vi "Common Function.vi"(6 "exit sig":refnum<k4>, 11 "gController in":refnum<class "gController.lvclass">) -> ()   [LabVIEW 2017, in "Controller.lvlib" / "gController.lvclass"]
uses:
  gController.lvclass
  C:/Program Files (x86)/National Instruments/LabVIEW 2017/vi.lib/MSR Consulting, LLC/General Reuse/SuperActor/SuperActor.lvclass
  C:/Program Files (x86)/National Instruments/LabVIEW 2017/vi.lib/ActorFramework/Actor/Actor.lvclass
  <vilib>/Platform/TimedLoop/XDataNode/timing_clust.ctl
  <vilib>/Platform/TimedLoop/XDataNode/nitl_modes.ctl
  <vilib>/Platform/TimedLoop/XDataNode/wakeup.ctl
  gController.lvclass/gController.ctl
  <vilib>/MSR Consulting, LLC/General Reuse/SuperActor/SuperActor.lvclass/SuperActor.ctl
  <vilib>/ActorFramework/Actor/Actor.lvclass/Actor.ctl
  <vilib>/ActorFramework/Message Enqueuer/Message Enqueuer.lvclass/Message Enqueuer.ctl
  <vilib>/MSR Consulting, LLC/General Reuse/Data/Data.lvclass/Data.ctl
  Messages/Update Controller Data MSG/Update gController Data MSG.lvclass
  C:/Program Files (x86)/National Instruments/LabVIEW 2017/vi.lib/MSR Consulting, LLC/General Reuse/Generic Update Data MSG/Generic Update Data MSG.lvclass
  C:/Program Files (x86)/National Instruments/LabVIEW 2017/vi.lib/ActorFramework/Message/Message.lvclass
  Data/SOAP Data.lvclass/SOAP Data.ctl
  <vilib>/MSR Consulting, LLC/General Reuse/Generic Update Data MSG/Generic Update Data MSG.lvclass/Generic Update Data MSG.ctl
  Data/Write temperatures.vi
  Data/Write interlock.vi
  Data/Read message_data.vi
  <vilib>/MSR Consulting, LLC/General Reuse/Generic Update Data MSG/Write Data.vi
  <vilib>/MSR Consulting, LLC/General Reuse/Generic Update Data MSG/Write ID.vi
  Read FPGA Session.vi
  <vilib>/MSR Consulting, LLC/General Reuse/SuperActor/Read Log Session.vi
  <vilib>/MSR Consulting, LLC/General Reuse/SuperActor/Read CVT Session.vi
  <vilib>/MSR Consulting, LLC/General Reuse/Data/Write write time.vi
  <vilib>/ActorFramework/Message Enqueuer/Init from Existing Queue.vi
  Session/Raw FPGA/FPGA Session.lvclass
  C:/Program Files (x86)/National Instruments/LabVIEW 2017/vi.lib/MSR Consulting, LLC/General Reuse/Session APIs/_Session Fwk/Session - Root.lvclass
  Data/SOAP Data.lvclass
  C:/Program Files (x86)/National Instruments/LabVIEW 2017/vi.lib/MSR Consulting, LLC/General Reuse/Data/Data.lvclass
  Global DO.vi
  <vilib>/Utility/error.llb/Error Cluster From Error Code.vi
  <vilib>/rvi/errors/niLvFpgaAdjustHostInterfaceError.vi
  <vilib>/MSR Consulting, LLC/General Reuse/Data/Write measTime.vi
  <vilib>/ActorFramework/Message Priority Queue/Priority Enqueue.vi
  <vilib>/MSR Consulting, LLC/General Reuse/Session APIs/_Session Fwk/Session - Root.lvclass
  <vilib>/ActorFramework/Message Enqueuer/Message Enqueuer.lvclass
  <vilib>/Platform/TimedLoop/XDataNode/XDataNode.xnode
  Data/Heater Data/Heater Data.lvclass
  <vilib>/rvi/interface/nirviReadWriteControl/nirviReadWriteControl.xnode
  FPGA Ref.ctl
  FPGA Bitfiles/server.lvbitx
  <vilib>/MSR Consulting, LLC/General Reuse/SuperActor/SuperActor.lvclass
  <vilib>/Platform/TimedLoop/XDataNode/XDNodeRunTimeDep.lvlib
  <vilib>/MSR Consulting, LLC/General Reuse/Session APIs/Session Log/System Log.lvclass
  <vilib>/ActorFramework/Actor/Actor.lvclass
  NiFpgaLv.dll
  <vilib>/MSR Consulting, LLC/General Reuse/Session APIs/CVT/CVT.lvclass
panel:
  out "Iteration Duration":i64
  out "exceeds_dead_line":bool
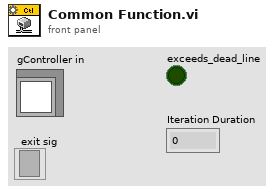
[diagram p1: front panel]
types:
  T1 = typedef "Session - Root.lvclass/Session Handle.ctl" = refnum<data-value>
  T2 = typedef "FPGA Ref.ctl" = refnum<k20>
  T3 = typedef "XDNodeRunTimeDep.lvlib/timing_clust.ctl" = cluster{"Expected End [f-1]":u64, "Actual End [f-1]":u64, "Finished Late? [f-1]":bool, "Expected End [i-1]":u64, "Actual End [i-1]":u64, "Finished Late? [i-1]":bool, "Expected Start [i]":u64, "Actual Start [i]":u64, "Expected Start [f]":u64, "Actual Start [f]":u64, "Source Name":string, "Structure Name":string, "Period":i64, "Deadline":i64, "Offset":i64, "Start":i64, "Priority":i32, "Timeout":i32, "Mode":T4, "Wakeup Reason":T5, "Error":errorcluster, "Source Type":string, "Secondary Source Type":string, "Global End Time":u64, "Global Start Time":u64, "Frame Duration":u64, "Iteration Duration":u64, "Assigned CPU":i32, "I/O Scan Engine Mode":u32}
  T4 = typedef "XDNodeRunTimeDep.lvlib/nitl_modes.ctl" = enum32{"No Change", "Process missed periods, maintain original phase", "Discard missed periods, maintain original phase", "Process missed periods, ignore original phase", "Discard missed periods, ignore original phase"}
  T5 = typedef "XDNodeRunTimeDep.lvlib/wakeup.ctl" = enum32{"Normal", "Aborted", "Asynchronous wakeup", "Timing source error", "Timed loop error", "Timeout"}
  T6 = cluster{"PAS Cell 1 Temperature":fxp<+/-,24,-2>, "PAS Cell 2 Temperature":fxp<+/-,24,-2>, "PAS Laser Head 1 Temperature":fxp<+/-,24,-2>, "PAS Laser Head 2 Temperature":fxp<+/-,24,-2>, "CRD Laser Head Temperature":fxp<+/-,24,-2>, "Box In Temperature":fxp<+/-,24,-2>, "Box Exit Temperature":fxp<+/-,24,-2>, "CRD Heater Temperature":fxp<+/-,24,-2>, "CJC":fxp<+/-,24,-2>, "Autozero":fxp<+/-,24,-2>}
  T7 = cluster{"PAS Cell 1 Temperature":dbl, "PAS Cell 2 Temperature":dbl, "PAS Laser Head 1 Temperature":dbl, "PAS Laser Head 2 Temperature":dbl, "CRD Laser Head Temperature":dbl, "Box In Temperature":dbl, "Box Exit Temperature":dbl, "CRD Heater Temperature":dbl, "CJC":dbl, "Autozero":dbl}
  T8 = cluster{"Temperature[0]":dbl, "Temperature[1]":dbl, "Temperature[2]":dbl, "Temperature[3]":dbl, "Temperature[4]":dbl, "Temperature[5]":dbl, "Temperature[6]":dbl, "Temperature[7]":dbl, "Temperature[8]":dbl, "Temperature[9]":dbl}
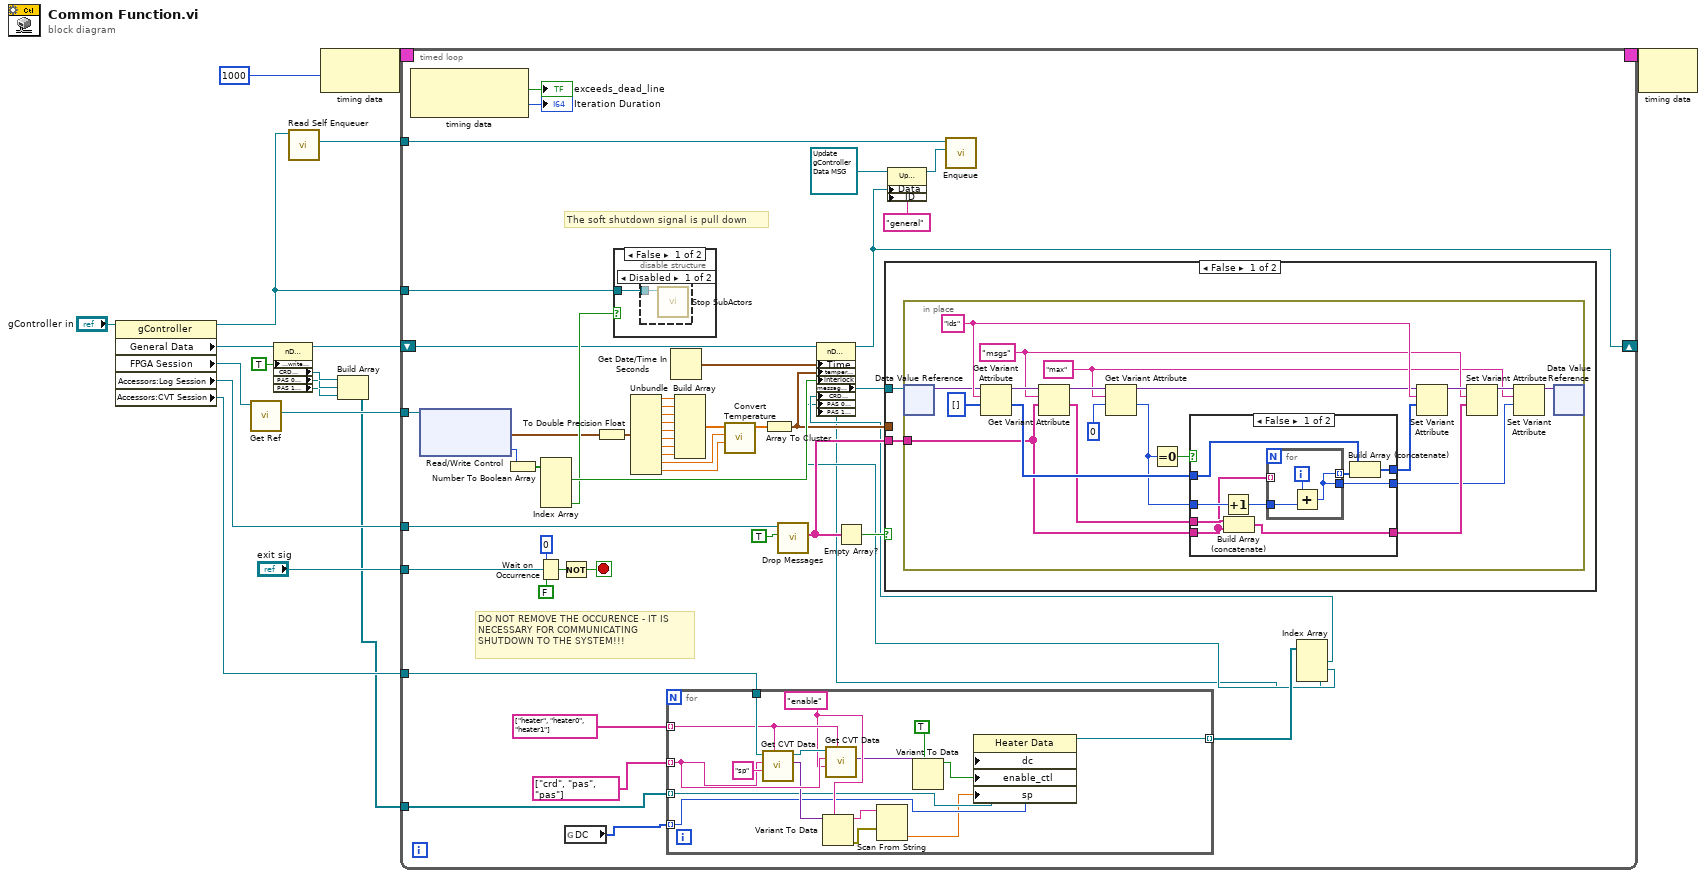
[diagram p0: block diagram]
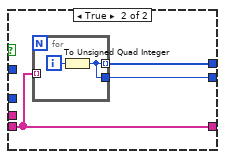
[diagram p2: hidden frame]
diagram:
  n1 = property class="gController"(reference="gController in") -> (reference out=w13:refnum<class "gController.lvclass">, "General Data"=w8:refnum<class "SOAP Data.lvclass">, "FPGA Session"=w10:refnum<data-value>, "Accessors:Log Session"=w9:T1, "Accessors:CVT Session"=w5:T1)  [unwired: 1 in, 1 out]
  n2 = call "Get Ref.vi"("Hanlde Out"=w10) -> ("FPGA Ref"=w14:T2)  [unwired: 8 in, 2 out]
  n3 = property class="nData"(reference=w8, "Accessors:write time"=TRUE ("write time")) -> (reference out=w7:refnum<class "SOAP Data.lvclass">, "CRD Heater"=w4:refnum<class "Heater Data.lvclass">, "PAS 0 Heater"=w3:refnum<class "Heater Data.lvclass">, "PAS 1 Heater"=w2:refnum<class "Heater Data.lvclass">)  [unwired: 1 in, 1 out]
  n4 = call <vilib>:"Read Self Enqueuer.vi"("Actor"=w13) -> ("Self Enqueuer"=w12:refnum<class "Message Enqueuer.lvclass">)  [unwired: 10 in]
  n5 = node-c288(i64 1000 ("Period")) -> (w18:T3)
  n6 = Build Array(w4, w3, w2) -> (w1:refnum<class "Heater Data.lvclass">[])
  n7 = timed-loop {
    tunnel: w14 -> [w67]
    timing: w18 -> [_]
    timing-out: [_] -> w17
    tunnel: w13 -> [w66]
    tunnel: w9 -> [w65]
    shift-right: [w53] -> _
    shift-left: w7 -> [w31]
    tunnel: w12 -> [w56]
    tunnel: "exit sig" -> [w49]
    tunnel: w5 -> [w25]
    tunnel: w1 -> [w23]
    stop <- w45 stop-if-true
    # "The soft shutdown signal is pull down"
    # "DO NOT REMOVE THE OCCURENCE - IT IS NECESSARY FOR COMMUNICATING SHUTDOWN TO THE SYSTEM!!!"
    n8 = node-c288() -> (→"exceeds_dead_line":bool, →"Iteration Duration":i64)  [unwired: 1 in]
    n9 = xnode "Read/Write Control"("FPGA VI Reference In"=w67) -> ("Temperatures"=w29:T6, "Sensor Status"=w30:u8)  [unwired: 1 in, 2 out]
    n10 = Number To Boolean Array(number=w30) -> (Boolean array=w50:bool[])
    n11 = Wait on Occurrence(1:FALSE ("ignore previous (T)"), 2:w49, 3:0 ("ms timeout (-1)")) -> (0:w46:bool)
    n12 = Index Array(array=w50) -> (element #1=w62:bool, element #4=w44:bool)  [unwired: 4 in, 2 out]
    n13 = Not(x=w46) -> (.not. x?=w45:bool)
    n14 = global read "Global DO.vi" "DC"() -> (w24:u8[])
    n15 = To Double Precision Float(number=w29) -> (double precision float=w39:T7)
    n16 = case shown="False" w44 {
      tunnel: w66 -> [w126 _]
      frame False {
        n17 = disable-structure shown="Disabled" {
          disable-tunnel: w126 -> [w127 _]
          frame Disabled {
            n18 = call <vilib>:"Stop SubActors.vi"("SuperActor in"=w127) -> ()  [unwired: 10 in, 1 out]
          }
          frame Enabled {
          }
        }
      }
      frame True {
      }
    }
    n19 = Unbundle(w39) -> ("PAS Cell 1 Temperature"=w43:dbl, "PAS Cell 2 Temperature"=w42:dbl, "PAS Laser Head 1 Temperature"=w41:dbl, "PAS Laser Head 2 Temperature"=w40:dbl, "CRD Laser Head Temperature"=w38:dbl, "Box In Temperature"=w37:dbl, "Box Exit Temperature"=w36:dbl, "CRD Heater Temperature"=w35:dbl, "CJC"=w33:dbl, "Autozero"=w32:dbl)
    n20 = for {
      tunnel: string[] ["crd", "pas", "pas"] -> [w79] mode=indexing
      tunnel: string[] ["heater", "heater0", "heater1"] -> [w80] mode=indexing
      tunnel: w25 -> [w83]
      tunnel: w24 -> [w71] mode=indexing
      tunnel: w23 -> [w72] mode=indexing
      tunnel: [w68] -> w22 mode=indexing
      w76 = "enable" ("Variable")
      n21 = call <vilib>:"Get CVT Data.vi"("Subgroup"=w80, "Variable"="sp", "Group"=w79, "CVT Session In"=w83) -> ("Data Out"=w77:variant, "CVT Session Out"=w81:T1)  [unwired: 4 in, 2 out]
      n22 = Variant To Data(type=w76, Variant=w77) -> (data=w75:string, error out=w78:errorcluster)  [unwired: 1 in]
      n23 = call <vilib>:"Get CVT Data.vi"("Subgroup"=w80, "Variable"=w76, "Group"=w79, "CVT Session In"=w81) -> ("Data Out"=w74:variant)  [unwired: 4 in, 3 out]
      n24 = Scan From String(input string=w75, error in=w78) -> (output 1=w69:dbl)  [unwired: 3 in, 3 out]
      n25 = Variant To Data(type=TRUE, Variant=w74) -> (data=w70:bool)  [unwired: 1 in, 1 out]
      n26 = property class="Heater Data"(reference=w72, "dc"=w71, "enable_ctl"=w70, "sp"=w69) -> (reference out=w68:refnum<class "Heater Data.lvclass">)  [unwired: 1 in, 1 out]
    }
    n27 = Get Date/Time In Seconds() -> (seconds since 1Jan1904=w61:timestamp)
    n28 = Build Array(w43, w42, w41, w40, w38, w37, w36, w35) -> (w34:dbl[])
    n29 = call "Convert Temperature.vi"("AutoZero"=w32, "CJC"=w33, "TC Input"=w34) -> ("Temperature"=w51:dbl[])  [unwired: 8 in]
    n30 = Array To Cluster(array=w51) -> (cluster=w28:T8)
    n31 = call <vilib>:"Drop Messages.vi"("Drop?"=TRUE, "log in"=w65) -> ("Current Msgs"=w58:string[])  [unwired: 7 in, 2 out]
    n32 = Empty Array?(array=w58) -> (empty?=w59:bool)
    n33 = Index Array(array=w22) -> (element #1=w21:refnum<class "Heater Data.lvclass">, element #2=w20:refnum<class "Heater Data.lvclass">, element #3=w19:refnum<class "Heater Data.lvclass">)  [unwired: 3 in]
    n34 = property class="nData"(reference=w31, "Time"=w61, "temperatures"=w28, "interlock"=w62, "CRD Heater"=w21, "PAS 0 Heater"=w20, "PAS 1 Heater"=w19) -> (reference out=w53:refnum<class "SOAP Data.lvclass">, "message_data"=w57:refnum<data-value>)  [unwired: 1 in, 1 out]
    n35 = case shown="False" w59 {
      tunnel: w58 -> [w85 _]
      tunnel: w57 -> [w84 _]
      tunnel: w28 -> [_ _]
      frame False {
        n36 = in-place {
          in-place-border: w85 -> [w101]
          w90 = "max" ("name")
          w98 = "msgs" ("name")
          w103 = "ids" ("name")
          n37 = in-place-dvr #1(w84) -> (w88:variant)  [unwired: 1 out]
          n38 = Get Variant Attribute(Variant=w88, name=w103, default value (empty Variant)=u64[] []) -> (duplicate Variant=w102:variant, value=w104:u64[])  [unwired: 1 in, 2 out]
          n39 = Get Variant Attribute(Variant=w102, name=w98, default value (empty Variant)=w101) -> (duplicate Variant=w95:variant, value=w100:string[])  [unwired: 1 in, 2 out]
          n40 = Get Variant Attribute(Variant=w95, name=w90, default value (empty Variant)=u64 0) -> (duplicate Variant=w93:variant, value=w91:u64)  [unwired: 1 in, 2 out]
          n41 = Equal To 0?(x=w91) -> (x = 0?=w92:bool)
          n42 = case shown="False" w92 {
            tunnel: w104 -> [w108 _]
            tunnel: [w106 w120] -> w86
            tunnel: w101 -> [w109 w119]
            tunnel: [w110 w119] -> w97
            tunnel: w100 -> [w111 _]
            tunnel: w91 -> [w114 _]
            tunnel: [w112 w118] -> w89
            frame False {
              n43 = Increment(x=w114) -> (x+1=w113:u64)
              n44 = Build Array (concatenate)(w111, w109) -> (w110:string[])
              n45 = for {
                tunnel: w113 -> [w116]
                tunnel: [w115] -> w107 mode=indexing
                tunnel: [w115] -> w112
                tunnel: w109 -> [_] mode=indexing
                i -> [w117]
                n46 = Add(x=w117, y=w116) -> (x+y=w115:u64)
              }
              n47 = Build Array (concatenate)(w108, w107) -> (w106:u64[])
            }
            frame True {
              n48 = for {
                tunnel: [w121] -> w120 mode=indexing
                tunnel: w119 -> [_] mode=indexing
                tunnel: [w121] -> w118
                i -> [w122]
                n49 = To Unsigned Quad Integer(1:w122) -> (0:w121:u64)
              }
            }
          }
          n50 = Set Variant Attribute(Variant=w93, name=w103, value=w86) -> (Variant out=w99:variant)  [unwired: 1 in, 2 out]
          n51 = Set Variant Attribute(Variant=w99, name=w98, value=w97) -> (Variant out=w96:variant)  [unwired: 1 in, 2 out]
          n52 = Set Variant Attribute(Variant=w96, name=w90, value=w89) -> (Variant out=w87:variant)  [unwired: 1 in, 2 out]
          n53 = in-place-dvr #1(w87) -> ()  [unwired: 2 out]
        }
      }
      frame True {
      }
    }
    n54 = property class="Update gController Data MSG.lvc"(reference=refnum<class "Update gController Data MSG.lvclass"> refnum ("Controller.lvlib:Update gController Data MSG.lvclass"), "Data"=w53, "ID"="general" ("name")) -> (reference out=w52:refnum<class "Update gController Data MSG.lvclass">)  [unwired: 1 in, 1 out]
    n55 = call <vilib>:"Enqueue.vi"("Message"=w52, "Message Enqueuer in"=w56) -> ()  [unwired: 8 in, 2 out]
  }
  n56 = node-c288(w17) -> ()  [unwired: 1 out]
